vi "UserFunctions.vi"() -> ()   [LabVIEW 2013]
panel:
  in  "User Functions":string="\n-- -------------------------------------------------------------------------------------------\n-- The following functions are part of the \"standard load\" of functions and should not be messed with\n-- They are here for reference only.\n-- Please add any user functions above this comment\n-- -------------------------------------------------------------------------------------------\n\n-- Creates a linear ramp from A to B\nfunction LineRamp(f, Initial, Final)\n    return (1-f)*Initial + f*Final;\nend\n\n-- Creates an exponential ramp from A to B\nfunction ExpRamp(t, a, b, tau)\n   return (b - a*exp(tMax / tau) + (a-b)*exp(t/tau))/ ( 1 - exp(tMax / tau) );\nend\n\n-- Creates a sinewave\nfunction SinRamp(t,Offset,A,Freq, Phase)\n    return Offset + A * sin(2*pi*Freq*t + Phase)\nend\n\n-- Creates a blackman pulse\nfunction Blackman(f, Offset, A)\n    return Offset +  A*sqrt(0.5*cos(3.1415*(2*f-1))+0.08*cos(2*pi*(2*f-1))+0.42);\nend\n\n-- Creates a half-gauss ramp\nfunction HalfGaussRamp(t, a, b, Width)\n    local y;\n    y = exp(-(tMax^2)/Width^2);\n    y = (a -  b*y)/(1-y)  +  ((b-a)/(1-y))*exp(-((t-tMax)^2)/Width^2);\n    return y;\nend"
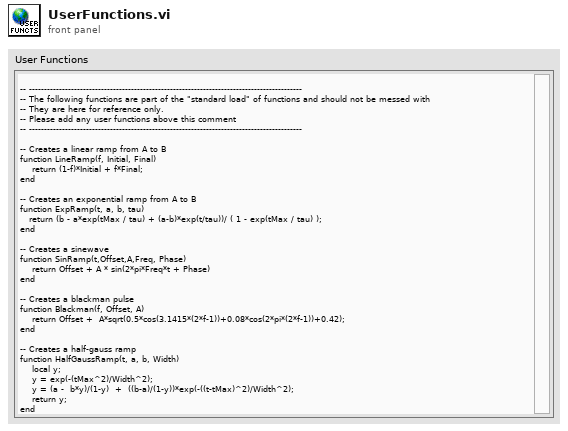
[diagram p1: front panel]
diagram:
